vi "Send Normal Stop.vi"(8 "error in (no error)":errorcluster, 11 "Message Enqueuer":refnum<class "Message Enqueuer.lvclass">) -> (0 "error out":errorcluster)   [LabVIEW 2017, in "Actor Framework.lvlib" / "Stop Msg.lvclass"]
doc: "(<B>Filename</B>: Actor Framework.lvlib:Stop Msg.lvclass:Send Normal Stop.vi)\n\nSends a Stop message to an actor, triggering the actor to run its Stop Core method. This message has normal priority, meaning the actor will process this message after processing high- or normal-priority messages that are in the queue already."
uses:
  Stop Msg.lvclass
  Message Enqueuer/Message Enqueuer.lvclass
  C:/LabVIEW Packages/Sources/PPLs/source/ActorFramework/Message/Message.lvclass
  Message Enqueuer/Message Enqueuer.lvclass/Message Enqueuer.ctl
  Message Priority Queue/Priority Enqueue.vi
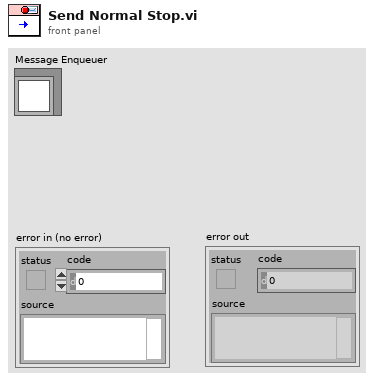
[diagram p1: front panel]
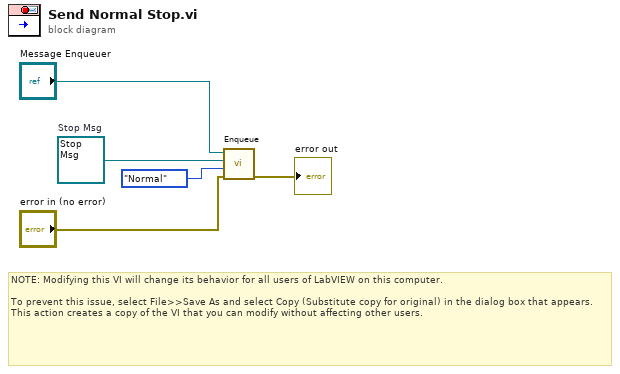
[diagram p0: block diagram]
diagram:
  w4 = refnum<class "Stop Msg.lvclass"> refnum  # Stop Msg
  # "NOTE: Modifying this VI will change its behavior for all users of LabVIEW on this computer.\n\nTo prevent this issue, select File>>Save As and select Copy (Substitute copy for original) in the dialog box that appears. This action creates a copy of the VI that you can modify without affecting other users."
  n1 = call "Enqueue.vi"("error in (no error)"="error in (no error)", "Message Priority (Normal)"=enum16{"Low", "Normal", "High"}."Normal" ("Queue Priority (Normal)"), "Message"=w4, "Message Enqueuer in"="Message Enqueuer") -> ("error out"=→"error out":errorcluster)  [unwired: 6 in, 1 out]
